vi "111.vi"() -> ()   [LabVIEW 2018]
uses:
  <vilib>/Utility/error.llb/DialogType.ctl
  <vilib>/DAQmx/read.llb/DAQmx Read (Analog 1D Wfm NChan NSamp).vi
  <vilib>/DAQmx/create/channels.llb/DAQmx Create Channel (AI-Voltage-Basic).vi
  <vilib>/DAQmx/configure/timing.llb/DAQmx Timing (Sample Clock).vi
  <vilib>/DAQmx/configure/task.llb/DAQmx Configure Logging (TDMS).vi
  <vilib>/DAQmx/configure/trigger.llb/DAQmx Start Trigger (Digital Edge).vi
  <vilib>/DAQmx/configure/trigger.llb/DAQmx Start Trigger (Time).vi
  <vilib>/DAQmx/configure/trigger.llb/DAQmx Start Trigger (Analog Edge).vi
  <vilib>/DAQmx/miscellaneous.llb/DAQmx Fill In Error Info.vi
  <vilib>/Waveform/WDTOps.llb/WDT Index Channel DBL.vi
  <resource>/objmgr/daqmx.rc
panel:
  in  "触发类型":T1(tab)
  in  "数字开始参考触发边沿":i32(ring)=10280 caption="边沿" items=["上升"=10280, "下降"=10171]
  in  "数字开始参考触发源":tag="/Dev1/PFI0" caption="源"
  in  "数字暂停触发暂停条件":i32(ring)=10192 caption="暂停条件" items=["高"=10192, "低"=10214]
  in  "数字暂停参考触发源":tag="/Dev1/PFI0" caption="源"
  in  "模拟开始触发基准":dbl caption="基准" format="%0.2f"
  in  "模拟开始触发滞后":dbl caption="滞后" format="%.2f"
  in  "模拟开始触发斜坡":i32(ring)=10280 caption="斜坡" items=["上升"=10280, "下降"=10171]
  in  "模拟开始触发源":string="APFI0" caption="源"
  in  "模拟暂停触发源":string="APFI0" caption="源"
  in  "模拟暂停触发暂停条件":i32(ring)=10093 caption="暂停条件" items=["高于基准"=10093, "低于基准"=10107]
  in  "模拟暂停触发基准":dbl caption="基准" format="%.2f"
  in  "发生条件":timestamp
  in  "手动选择\n时间":bool
  in  "停止":bool
  in  "TDMS文件路径":path
  in  "采样时钟源":tag="OnboardClock"
  in  "接线端配置":i32(ring)=-1 items=["默认"=-1, "RSE"=10083, "NRSE"=10078, "差分"=10106, "伪差分"=12529]
  in  "最大电压":dbl=5.0
  in  "最小电压":dbl=-5.0
  in  "物理通道":tag="Dev1/ai0"
  out "实际采样率":dbl=1000.0 format="%0.2f"
  in  "记录模式":i32(ring)=10231 items=["关"=10231, "记录并读取"=15842]
  # "要启用触发，选择上面的选项卡进行配置。\n\n有些硬件只支持部分触发类型。详细信息见设备的说明文档。"
  # "连续采样定时不支持该触发类型。\n\n关于设备支持的触发源的信息，见设备说明文档。"
  # "连续采样定时不支持该触发类型。\n\n关于设备支持的触发源的信息，见设备说明文档。"
  # "如未手动设置时间，任务将在10秒后开始"
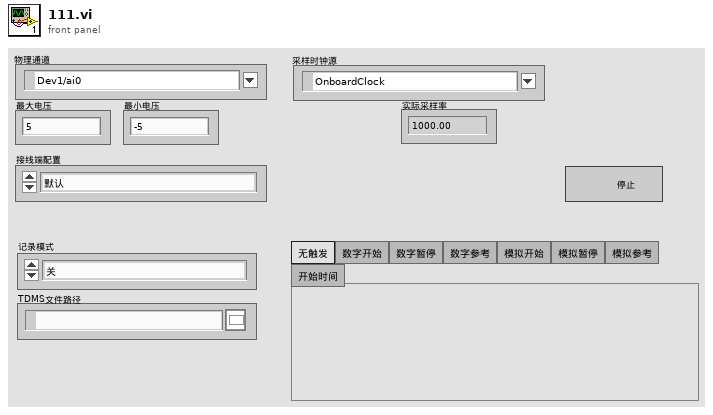
[diagram p1: front panel]
types:
  T1 = enum32{"No Trigger", "Digital Start", "Digital Pause", "Digital Reference", "Analog Start", "Analog Pause", "Analog Reference", "Time Start"}
  T2 = typedef "DialogType.ctl" = u16
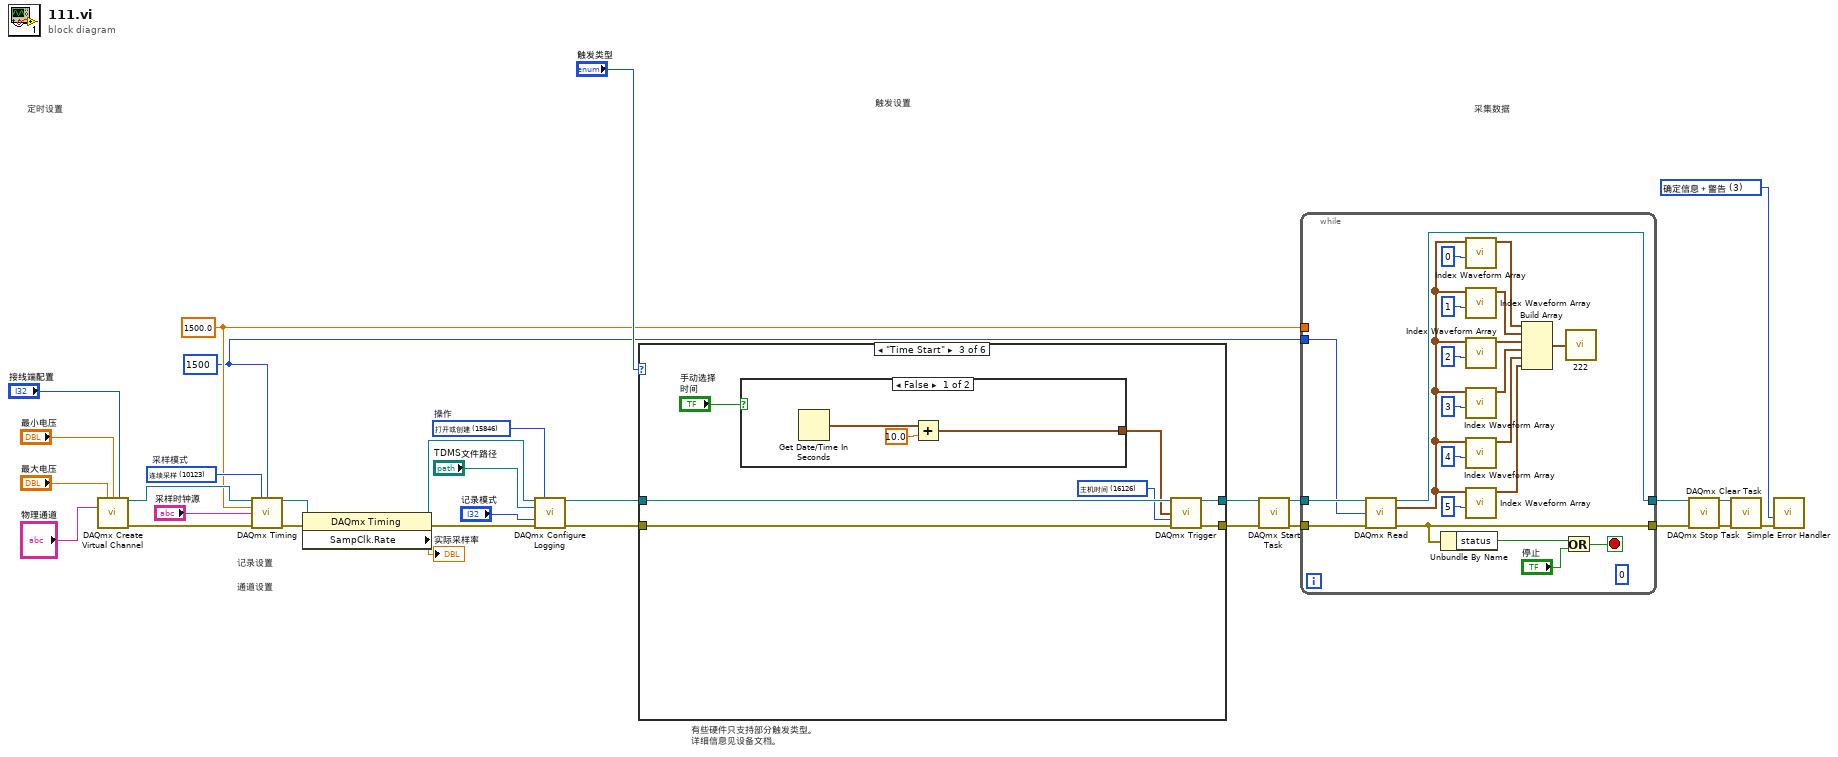
[diagram p0: block diagram]
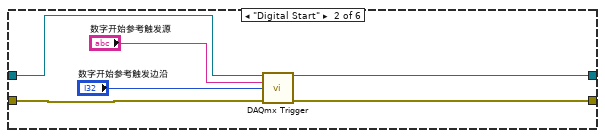
[diagram p3: hidden frame]
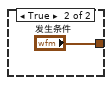
[diagram p4: hidden frame]
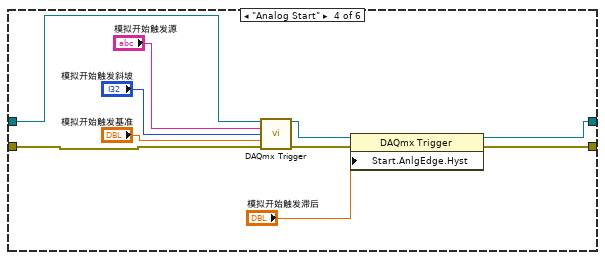
[diagram p5: hidden frame]
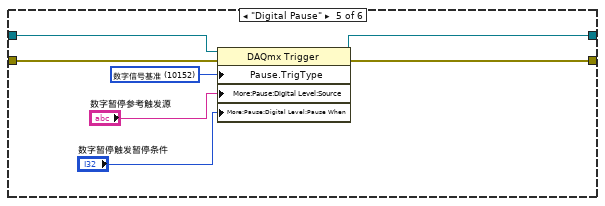
[diagram p6: hidden frame]
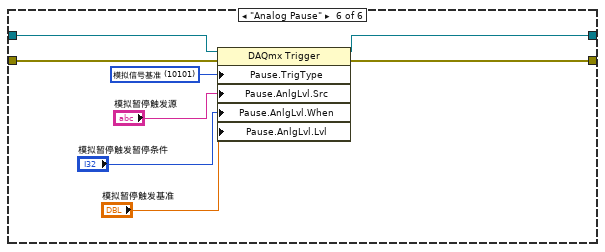
[diagram p7: hidden frame]
diagram:
  w1 = 1500 ("samples per channel")
  w2 = 1500.0 ("rate")
  w8 = T2 3 items=["无对话框", "确定信息", "继续或停止信息", "确定信息＋警告", "继续/停止＋警告"] ("对话框类型（确定信息：1）")
  w24 = 15846 items=["打开"=10437, "打开或创建"=15846, "创建或替换"=15847, "创建"=15848]  # 操作
  w29 = 10123 items=["有限采样"=10178, "连续采样"=10123, "硬件定时单点"=12522]  # 采样模式
  # "触发设置"
  # "有些硬件只支持部分触发类型。\n详细信息见设备文档。"
  # "采集数据"
  # "定时设置"
  # "通道设置"
  # "记录设置"
  n1 = call-poly <vilib>:"DAQmx Create Virtual Channel.vi"("maximum value"="最大电压", "minimum value"="最小电压", "input terminal configuration"="接线端配置", "physical channels"="物理通道") -> ("task out"=w27:refnum<k21>, "error out"=w28:errorcluster)  [unwired: 10 in]
  n2 = call-poly <vilib>:"DAQmx Timing.vi"("task/channels in"=w27, "sample mode"=w29, "samples per channel"=w1, "rate"=w2, "source"="采样时钟源", "error in"=w28) -> ("task out"=w31:refnum<k21>, "error out"=w30:errorcluster)  [unwired: 8 in]
  n3 = property class="DAQmx Timing"(reference=w31, error in=w30) -> (reference out=w26:refnum<k21>, error out=w25:errorcluster, "SampClk.Rate"=→"实际采样率":dbl)
  n4 = call-poly <vilib>:"DAQmx Configure Logging.vi"("task/channels in"=w26, "operation"=w24, "file path"="TDMS文件路径", "logging mode"="记录模式", "error in"=w25) -> ("task out"=w6:refnum<k21>, "error out"=w5:errorcluster)  [unwired: 9 in]
  n5 = case shown="\"Time Start\"" "触发类型" {
    tunnel: w6 -> [w33 w39 w46 w60 w67 w75]
    tunnel: w5 -> [w32 w38 w45 w59 w64 w72]
    tunnel: [w33 w37 w44 w57 w66 w74] -> w3
    tunnel: [w32 w36 w43 w56 w65 w73] -> w4
    frame "No Trigger", Default {
    }
    frame "Digital Start" {
      n6 = call-poly <vilib>:"DAQmx Trigger.vi"("task/channels in"=w39, "source"="数字开始参考触发源", "edge"="数字开始参考触发边沿", "error in"=w38) -> ("task out"=w37:refnum<k21>, "error out"=w36:errorcluster)  [unwired: 10 in]
    }
    frame "Time Start" {
      w42 = 16126 items=["主机时间"=16126, "I/O设备时间"=16127] ("时间缩放")
      n7 = case shown="False" "手动选择\n时间" {
        tunnel: [w47 "发生条件"] -> w40
        frame False {
          n8 = Get Date/Time In Seconds() -> (seconds since 1Jan1904=w49:timestamp)
          n9 = Add(x=w49, y=10.0) -> (x+y=w47:timestamp)
        }
        frame True {
        }
      }
      n10 = call-poly <vilib>:"DAQmx Trigger.vi"("task/channels in"=w46, "when"=w40, "timescale"=w42, "error in"=w45) -> ("task out"=w44:refnum<k21>, "error out"=w43:errorcluster)  [unwired: 10 in]
    }
    frame "Analog Start" {
      n11 = call-poly <vilib>:"DAQmx Trigger.vi"("task/channels in"=w60, "source"="模拟开始触发源", "slope"="模拟开始触发斜坡", "level"="模拟开始触发基准", "error in"=w59) -> ("task out"=w55:refnum<k21>, "error out"=w54:errorcluster)  [unwired: 9 in]
      n12 = property class="DAQmx Trigger"(reference=w55, error in=w54, "Start.AnlgEdge.Hyst"="模拟开始触发滞后") -> (reference out=w57:refnum<k21>, error out=w56:errorcluster)
    }
    frame "Digital Pause" {
      w63 = 10152 items=["模拟信号基准"=10101, "模拟窗"=10103, "数字信号基准"=10152, "数字模式"=10398, "无"=10230] ("暂停.触发类型")
      n13 = property class="DAQmx Trigger"(reference=w67, error in=w64, "Pause.TrigType"=w63, "More:Pause:Digital Level:Source"="数字暂停参考触发源", "More:Pause:Digital Level:Pause When"="数字暂停触发暂停条件") -> (reference out=w66:refnum<k21>, error out=w65:errorcluster)
    }
    frame "Analog Pause" {
      w71 = 10101 items=["模拟信号基准"=10101, "模拟窗"=10103, "数字信号基准"=10152, "数字模式"=10398, "无"=10230] ("暂停.触发类型")
      n14 = property class="DAQmx Trigger"(reference=w75, error in=w72, "Pause.TrigType"=w71, "Pause.AnlgLvl.Src"="模拟暂停触发源", "Pause.AnlgLvl.When"="模拟暂停触发暂停条件", "Pause.AnlgLvl.Lvl"="模拟暂停触发基准") -> (reference out=w74:refnum<k21>, error out=w73:errorcluster)
    }
  }
  n15 = call <vilib>:"DAQmx Start Task.vi"("task/channels in"=w3, "error in"=w4) -> ("task out"=w23:refnum<k21>, "error out"=w22:errorcluster)  [unwired: 12 in]
  n16 = while {
    tunnel: w23 -> [w97]
    tunnel: w22 -> [w96]
    tunnel: [w95] -> w12
    tunnel: [w93] -> w11
    tunnel: w1 -> [w90]
    tunnel: w2 -> [_]
    stop <- w91 stop-if-true
    (unwired) 0
    n17 = call-poly <vilib>:"DAQmx Read.vi"("task/channels in"=w97, "number of samples per channel"=w90, "error in"=w96) -> ("task out"=w95:refnum<k21>, "data"=w83:waveform(dbl)[], "error out"=w93:errorcluster)  [unwired: 10 in]
    n18 = Unbundle By Name(w93) -> ("status"=w92:bool)
    n19 = call-poly <vilib>:"Index Waveform Array.vi"("index"=0, "waveform array"=w83) -> ("waveform"=w82:waveform(dbl))  [unwired: 8 in, 1 out]
    n20 = call-poly <vilib>:"Index Waveform Array.vi"("index"=1, "waveform array"=w83) -> ("waveform"=w81:waveform(dbl))  [unwired: 8 in, 1 out]
    n21 = call-poly <vilib>:"Index Waveform Array.vi"("index"=2, "waveform array"=w83) -> ("waveform"=w80:waveform(dbl))  [unwired: 8 in, 1 out]
    n22 = call-poly <vilib>:"Index Waveform Array.vi"("index"=3, "waveform array"=w83) -> ("waveform"=w79:waveform(dbl))  [unwired: 8 in, 1 out]
    n23 = call-poly <vilib>:"Index Waveform Array.vi"("index"=4, "waveform array"=w83) -> ("waveform"=w78:waveform(dbl))  [unwired: 8 in, 1 out]
    n24 = call-poly <vilib>:"Index Waveform Array.vi"("index"=5, "waveform array"=w83) -> ("waveform"=w77:waveform(dbl))  [unwired: 8 in, 1 out]
    n25 = Build Array(w82, w81, w80, w79, w78, w77) -> (w76:waveform(dbl)[])
    n26 = Or(x=w92, y="停止") -> (x .or. y?=w91:bool)
    n27 = call "222.vi"("波形 I/Q 1"=w76) -> ()
  }
  n28 = call <vilib>:"DAQmx Stop Task.vi"("task/channels in"=w12, "error in"=w11) -> ("task out"=w9:refnum<k21>, "error out"=w10:errorcluster)  [unwired: 12 in]
  n29 = call <vilib>:"DAQmx Clear Task.vi"("task in"=w9, "error in"=w10) -> ("error out"=w21:errorcluster)  [unwired: 13 in]
  n30 = call <vilib>:"Simple Error Handler.vi"("type of dialog (OK msg:1)"=w8, "error in (no error)"=w21) -> ()  [unwired: 3 in, 5 out]
